vi "Set Report Footer Text.vi"(0 "report in":T1, 5 "left footer text":string, 7 "center footer text":string, 9 "right footer text":string, 11 "error in (no error)":errorcluster, 12 "HTML footer size":enum16{"H1", "H2", "H3", "H4", "H5", "H6", "H7"}(ring)=enum."H3") -> (4 "report out":T1, 15 "error out":errorcluster)   [LabVIEW 2017]
doc: "Sets the text of the report footer."
uses:
  <vilib>/Utility/NIReport.llb/Generate Report Object Reference.ctl
  <vilib>/Utility/NIReport.llb/NI_report.lvclass
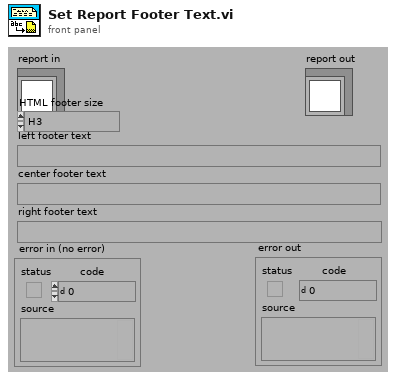
[diagram p1: front panel]
types:
  T1 = typedef "Generate Report Object Reference.ctl" = refnum<class "NI_report.lvclass">
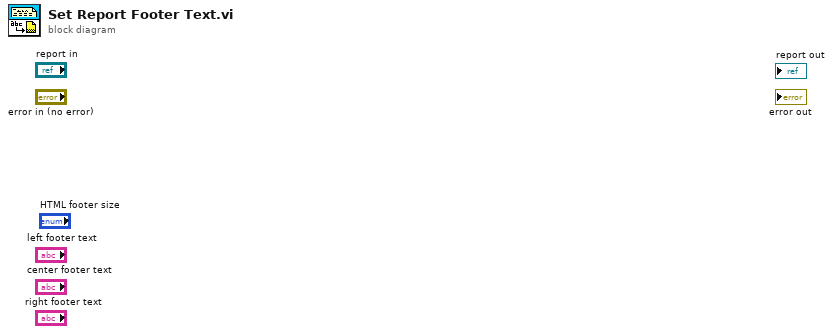
[diagram p0: block diagram]
diagram:
